vi "SFID_Open serial port.vi"(8 "Error in":errorcluster, 10 "timeout (ms)":u32=10000, 11 "VISA resource name":refnum<visa-resource-name>) -> (0 "Error out":errorcluster, 3 "VISA resource name out":refnum<visa-resource-name>)   [LabVIEW 2022 SP3]
uses:
  <vilib>/Instr/_visa.llb/VISA Open Access Mode.ctl
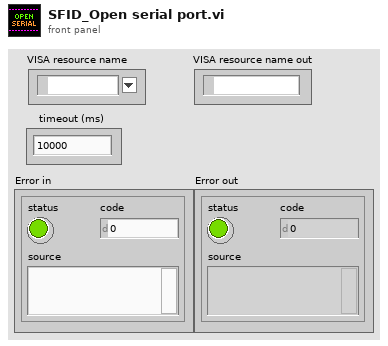
[diagram p1: front panel]
types:
  T1 = typedef "VISA Open Access Mode.ctl" = u32
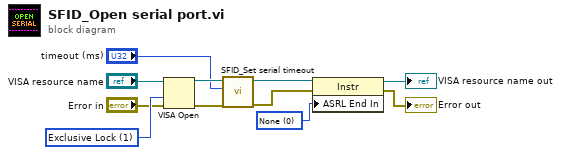
[diagram p0: block diagram]
diagram:
  w1 = u16 0 items=["None", "Last Bit", "TermChar"] ("Serial Settings:End Mode for Reads")
  w11 = T1 1 items=["VISA Defaults"=0, "Exclusive Lock"=1, "Load Configured Settings"=4] ("Access Mode")
  n1 = VISA Open(access mode=w11, error in (no error)="Error in", VISA resource name="VISA resource name") -> (VISA resource name=w5:refnum<visa-resource-name>, error out=w6:errorcluster)  [unwired: 2 in]
  n2 = call "SFID_Set serial timeout.vi"("Error In"=w6, "timeout (ms)"="timeout (ms)", "VISA resource name"=w5) -> ("Error Out"=w3:errorcluster, "VISA resource name out"=w4:refnum<visa-resource-name>)  [unwired: 7 in]
  n3 = property class="Instr"(reference=w4, error in=w3, "ASRL End In"=w1) -> (reference out=→"VISA resource name out":refnum<visa-resource-name>, error out=→"Error out":errorcluster)
